vi "Run Elevated.vi"(8 "error in (no error)":errorcluster, 11 "Script or EXE Path":path) -> (0 "error out":errorcluster)   [LabVIEW 2019, in "Tools.lvlib"]
doc: "This VI runs file of given <b>Script or EXE Path</b> with administrator privileges. For instance, if there is a command that needs to be elevated, you can use this VI instead of System Exec.vi - all you need to do is to prepare a .bat or .cmd file with the command and provide it as a VI input."
uses:
  Tools.lvlib
  shell32.dll
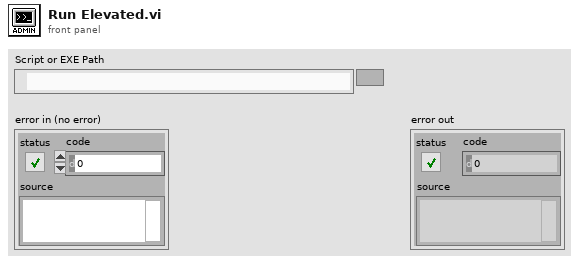
[diagram p1: front panel]
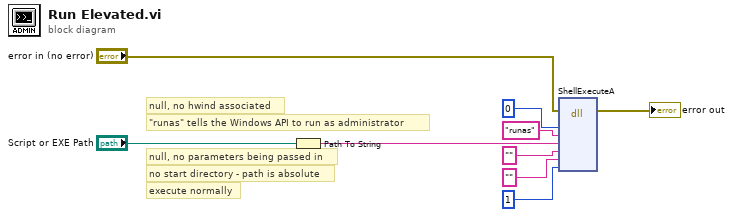
[diagram p0: block diagram]
diagram:
  # "no start directory - path is absolute"
  # "null, no parameters being passed in"
  # "null, no hwind associated"
  # "execute normally"
  # "\"runas\" tells the Windows API to run as administrator"
  n1 = Path To String(path="Script or EXE Path") -> (string=w3:string)
  n2 = dll-call lib="shell32.dll" fn="ShellExecuteA"(error in="error in (no error)", "hWnd"=0, "lpOperation"="runas", "lpFile"=w3, "lpParameters"="", "lpDirectory"="", "nShowCmd"=1) -> (error out=→"error out":errorcluster)  [unwired: 9 in, 1 out]
